vi "NI Read XLSX File.vi"(8 "error in":errorcluster, 11 "XLSX File":path) -> (0 "error out":errorcluster, 2 "Sheet Names":string[](array[string]), 3 "Sheet Data":cluster{"Array":string[][]}[](array[cluster]))   [LabVIEW 2018]
doc: "Reads all sheets from the specified <b>XLSX File</b>. This VI does <b>not</b> require Microsoft Excel to be installed.\n\nEach sheet is returned as a 2D Array of Strings. You will need to perform additional conversion if you require data in numeric format.\n\nTime data (date and/or time) is returned as a number of days elapsed since January 1, 1900. Hour/minute/second information will be returned as a fraction of a day (24 hours)."
uses:
  <vilib>/zip/NI_Unzip.lvlib
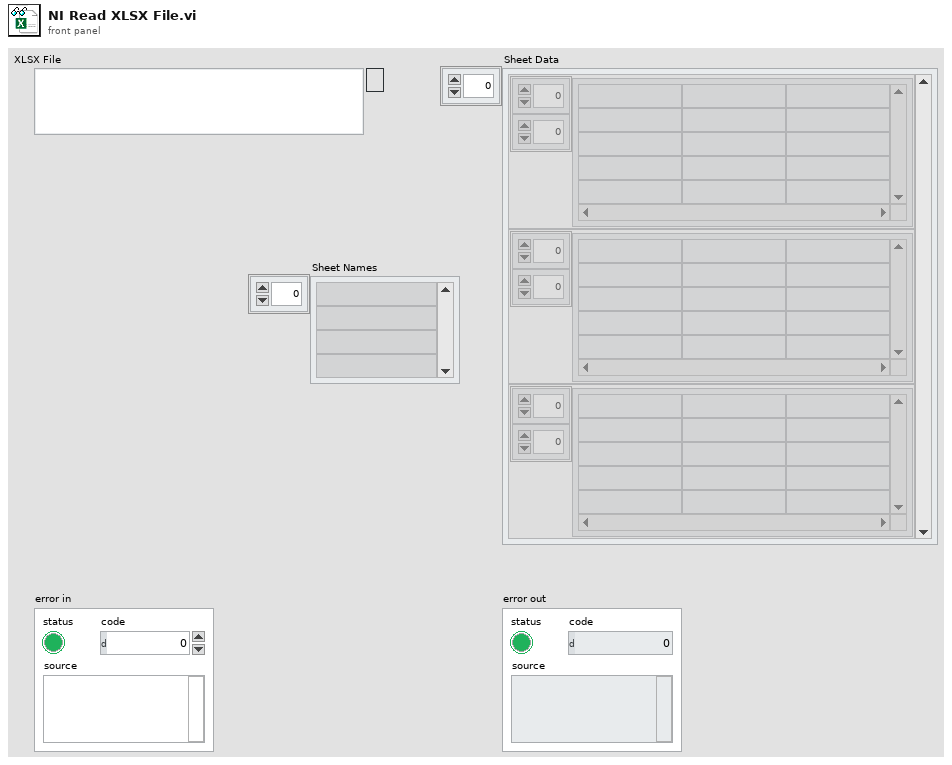
[diagram p1: front panel]
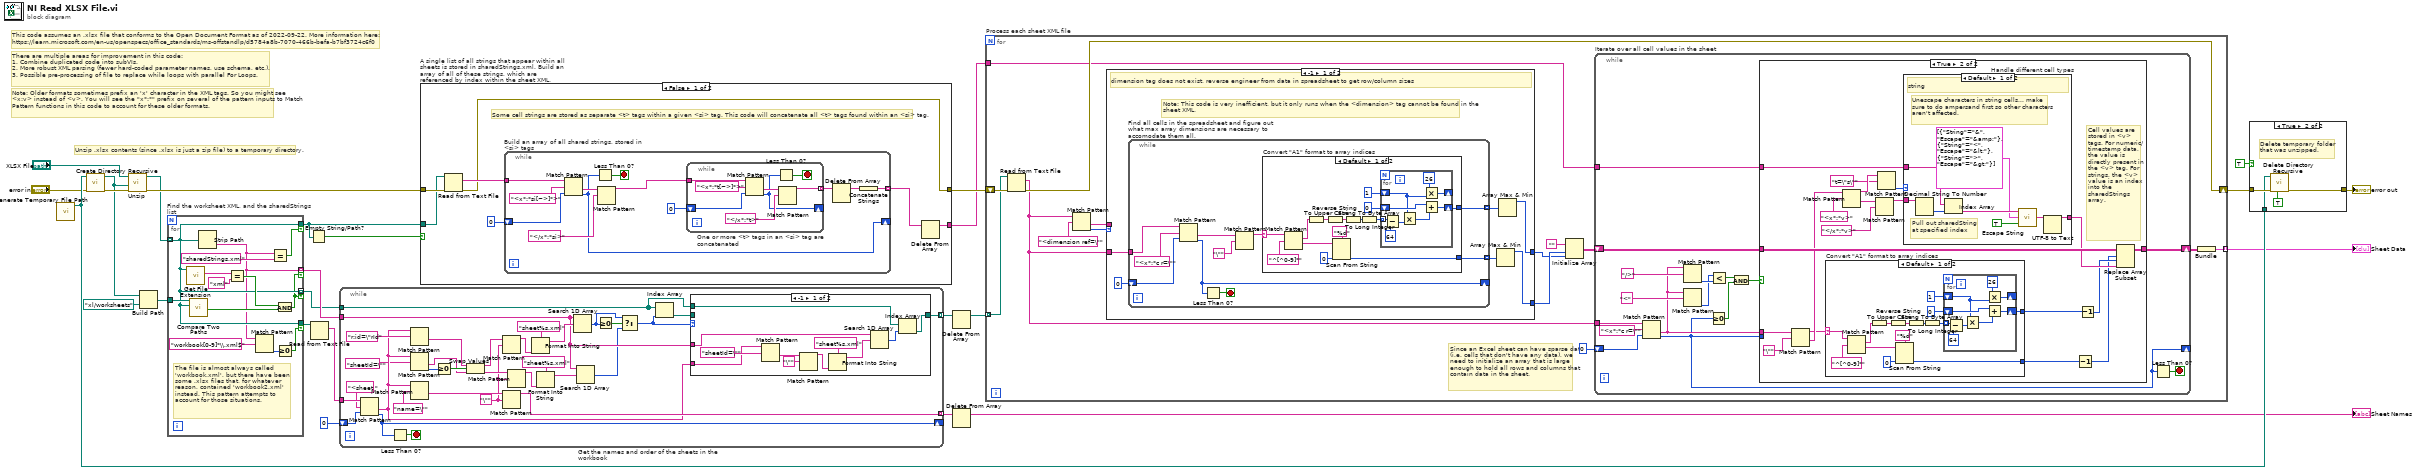
[diagram p0: block diagram]
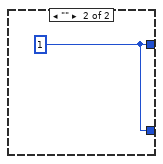
[diagram p5: hidden frame]
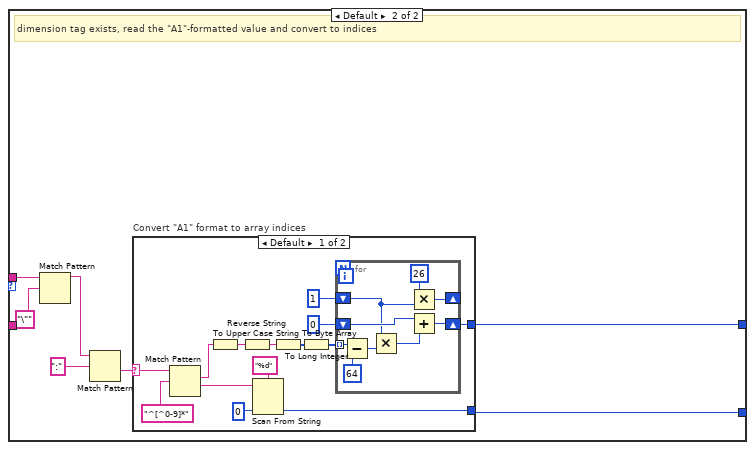
[diagram p6: hidden frame]
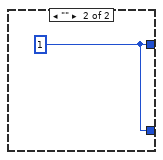
[diagram p7: hidden frame]
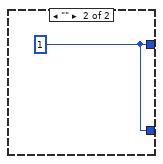
[diagram p9: hidden frame]
diagram:
  # "Note: Older formats sometimes prefix an 'x' character in the XML tags. So you might see <x:v> instead of <v>. You will see the \"x*:*\" prefix on several of the pattern inputs to Match Pattern functions in this code to account for these older formats."
  # "There are multiple areas for improvement in this code:\n1. Combine duplicated code into subVIs.\n2. More robust XML parsing (fewer hard-coded parameter names, use schema, etc.).\n3. Possible pre-processing of file to replace while loops with parallel For Loops."
  # "Unzip .xlsx contents (since .xlsx is just a zip file) to a temporary directory."
  # "This code assumes an .xlsx file that conforms to the Open Document Format as of 2022-09-22. More information here:\nhttps://learn.microsoft.com/en-us/openspecs/office_standards/ms-offstandlp/d5784a8b-7070-466b-befa-b7bf3724c6f0"
  n1 = call <vilib>:"Generate Temporary File Path.vi"() -> ("Unique Temporary File Path"=w16:path)  [unwired: 10 in, 1 out]
  n2 = call <vilib>:"Create Directory Recursive.vi"("error in (no error)"="error in", "directory"=w16) -> ("error out"=w26:errorcluster, "directory copy"=w19:path)  [unwired: 3 in, 1 out]
  n3 = call <vilib>:"Unzip.vi"("error in (no error)"=w26, "Target directory (same as Zip file if empty)"=w19, "Zip file"="XLSX File") -> ("error out"=w25:errorcluster, "Unzipped files"=w20:path[])  [unwired: 6 in, 1 out]
  n4 = Build Path(base path=w19, name or relative path=path "xl/worksheets") -> (appended path=w17:path)
  n5 = for "Find the worksheet XML, and the sharedStrings list" {
    tunnel: w20 -> [w32] mode=indexing
    tunnel: [w32] -> w13 if=w36
    tunnel: w17 -> [w38]
    tunnel: [w32] -> w7 mode=indexing if=w31
    tunnel: [w32] -> w11 if=w27
    tunnel: [w30] -> w8 mode=indexing if=w31
    # "The file is almost always called 'workbook.xml', but there have been some .xlsx files that, for whatever reason, contained 'workbook2.xml' instead. This pattern attempts to account for those situations."
    n6 = call <vilib>:"Get File Extension.vi"("file"=w32) -> ("lowercase file extension"=w35:string)  [unwired: 6 in, 4 out]
    n7 = call <vilib>:"Compare Two Paths.vi"("Path 2"=w32, "Path 1"=w38) -> ("Path 2 Relative to Path 1?"=w37:bool)  [unwired: 6 in, 3 out]
    n8 = Strip Path(path=w32) -> (name=w30:string)  [unwired: 1 out]
    n9 = Equal?(x=w35, y="xml") -> (x = y?=w33:bool)
    n10 = Match Pattern(string=w30, regular expression="workbook[0-9]*\\.xml$" ("y")) -> (offset past match=w28:i32)  [unwired: 1 in, 3 out]
    n11 = Equal?(x=w30, y="sharedStrings.xml") -> (x = y?=w36:bool)
    n12 = And(x=w33, y=w37) -> (x .and. y?=w31:bool)
    n13 = Greater Or Equal To 0?(x=w28) -> (x >= 0?=w27:bool)
  }
  n14 = Empty String/Path?(string/path=w13) -> (empty?=w12:bool)
  n15 = Read from Text File(file (use dialog)=w11) -> (text=w10:string)  [unwired: 3 in, 3 out]
  n16 = while "Get the names and order of the sheets in the workbook" {
    tunnel: w10 -> [w71]
    shift-right: [w69] -> _
    shift-left: 0 -> [w70]
    tunnel: [w63] -> w4 mode=indexing
    tunnel: w8 -> [w44]
    tunnel: w7 -> [w57]
    tunnel: [w59] -> w6 mode=indexing
    stop <- w67 stop-if-true
    w46 = "\"" ("regular expression")
    n17 = Match Pattern(string=w71, regular expression="<sheet ", offset (0)=w70) -> (after substring=w56:string, offset past match=w69:i32)  [unwired: 2 out]
    n18 = Less Than 0?(x=w69) -> (x < 0?=w67:bool)
    n19 = Match Pattern(string=w56, regular expression="r:id=\"rId") -> (after substring=w49:string)  [unwired: 1 in, 3 out]
    n20 = Match Pattern(string=w56, regular expression="name=\"") -> (after substring=w65:string)  [unwired: 1 in, 3 out]
    n21 = Match Pattern(string=w56, regular expression="sheetId=\"") -> (after substring=w50:string, offset past match=w54:i32)  [unwired: 1 in, 2 out]
    n22 = Greater Or Equal To 0?(x=w54) -> (x >= 0?=w51:bool)
    n23 = Swap Values(12:w49, 13:w51, 14:w50) -> (1:w48:string, 3:w47:string)
    n24 = Match Pattern(string=w48, regular expression=w46) -> (before substring=w62:string)  [unwired: 1 in, 3 out]
    n25 = Match Pattern(string=w65, regular expression=w46) -> (before substring=w63:string)  [unwired: 1 in, 3 out]
    n26 = Match Pattern(string=w47, regular expression=w46) -> (before substring=w52:string)  [unwired: 1 in, 3 out]
    n27 = Format Into String(format string="sheet%s.xml", w62) -> (resulting string=w60:string)  [unwired: 2 in, 1 out]
    n28 = Format Into String(format string="sheet%s.xml", w52) -> (resulting string=w45:string)  [unwired: 2 in, 1 out]
    n29 = Search 1D Array(1D array=w44, element=w60) -> (index of element=w42:i32)  [unwired: 1 in]
    n30 = Search 1D Array(1D array=w44, element=w45) -> (index of element=w41:i32)  [unwired: 1 in]
    n31 = Greater Or Equal To 0?(x=w42) -> (x >= 0?=w43:bool)
    n32 = Select(t=w42, s=w43, f=w41) -> (s? t:f=w40:i32)
    n33 = Index Array(array=w57, index=w40) -> (element=w58:path)
    n34 = case shown="-1" w40 {
      tunnel: [w76 w83] -> w59
      tunnel: w58 -> [_ w83]
      tunnel: w57 -> [w75 _]
      tunnel: w44 -> [w74 _]
      tunnel: w56 -> [w72 _]
      frame -1 {
        n35 = Match Pattern(string=w72, regular expression="sheetId=\"") -> (after substring=w81:string)  [unwired: 1 in, 3 out]
        n36 = Match Pattern(string=w81, regular expression="\"") -> (before substring=w80:string)  [unwired: 1 in, 3 out]
        n37 = Format Into String(format string="sheet%s.xml", w80) -> (resulting string=w78:string)  [unwired: 2 in, 1 out]
        n38 = Search 1D Array(1D array=w74, element=w78) -> (index of element=w77:i32)  [unwired: 1 in]
        n39 = Index Array(array=w75, index=w77) -> (element=w76:path)
      }
      frame Default {
      }
    }
  }
  n40 = case "A single list of all strings that appear within all sheets is stored in sharedStrings.xml. Build an array of all of these strings, which are referenced by index within the sheet XML." shown="False" w12 {
    tunnel: w25 -> [w90 w111]
    tunnel: [w85 w111] -> w24
    tunnel: w13 -> [w89 _]
    tunnel: [w86 _] -> w14
    frame False {
      # "Some cell strings are stored as separate <t> tags within a given <si> tag. This code will concatenate all <t> tags found within an <si> tag."
      n41 = Read from Text File(file (use dialog)=w89, error in=w90) -> (text=w88:string, error out=w85:errorcluster)  [unwired: 2 in, 2 out]
      n42 = while "Build an array of all shared strings, stored in <si> tags" {
        tunnel: w88 -> [w94]
        tunnel: [w99] -> w87 mode=indexing
        shift-right: [w93] -> _
        shift-left: 0 -> [w95]
        stop <- w91 stop-if-true
        n43 = Match Pattern(string=w94, regular expression="<x*:*si[~>]*>", offset (0)=w95) -> (after substring=w97:string, offset past match=w93:i32)  [unwired: 2 out]
        n44 = Less Than 0?(x=w93) -> (x < 0?=w91:bool)
        n45 = Match Pattern(string=w97, regular expression="</x*:*si>") -> (before substring=w92:string)  [unwired: 1 in, 3 out]
        n46 = while "One or more <t> tags in an <si> tag are concatenated" {
          tunnel: w92 -> [w110]
          tunnel: [w106] -> w102 mode=indexing
          shift-right: [w104] -> _
          shift-left: 0 ("offset past match") -> [w103]
          stop <- w105 stop-if-true
          n47 = Match Pattern(string=w110, regular expression="<x*:*t[~>]*>", offset (0)=w103) -> (after substring=w108:string, offset past match=w104:i32)  [unwired: 2 out]
          n48 = Less Than 0?(x=w104) -> (x < 0?=w105:bool)
          n49 = Match Pattern(string=w108, regular expression="</x*:*t>") -> (before substring=w106:string)  [unwired: 1 in, 3 out]
        }
        n50 = Delete From Array(array=w102) -> (array with subset deleted=w100:string[])  [unwired: 2 in, 1 out]
        n51 = Concatenate Strings(w100) -> (w99:string)
      }
      n52 = Delete From Array(array=w87) -> (array with subset deleted=w86:string[])  [unwired: 2 in, 1 out]
    }
    frame True {
      # "No sharedStrings.xml file within .xlsx."
    }
  }
  n53 = Delete From Array(array=w6) -> (array with subset deleted=w5:path[])  [unwired: 2 in, 1 out]
  n54 = Delete From Array(array=w4) -> (array with subset deleted=→"Sheet Names":string[])  [unwired: 2 in, 1 out]
  n55 = for "Process each sheet XML file" {
    shift-right: [w125] -> w23
    shift-left: w24 -> [w126]
    tunnel: w5 -> [w124] mode=indexing
    tunnel: [w118] -> w15 mode=indexing
    tunnel: w14 -> [w116]
    # "Since an Excel sheet can have sparse data (i.e. cells that don't have any data), we need to initialize an array that is large enough to hold all rows and columns that contain data in the sheet."
    n56 = Read from Text File(file (use dialog)=w124, error in=w126) -> (text=w112:string, error out=w125:errorcluster)  [unwired: 2 in, 2 out]
    n57 = Match Pattern(string=w112, regular expression="<dimension ref=\"") -> (after substring=w122:string, offset past match=w113:i32)  [unwired: 1 in, 2 out]
    n58 = case shown="-1" w113 {
      tunnel: w122 -> [_ w173]
      tunnel: [w129 w171] -> w115
      tunnel: [w127 w170] -> w114
      tunnel: w112 -> [w132 _]
      frame -1 {
        # "Note: This code is very inefficient, but it only runs when the <dimension> tag cannot be found in the sheet XML."
        # "dimension tag does not exist, reverse engineer from data in spreadsheet to get row/column sizes"
        n59 = while "Find all cells in the spreadsheet and figure out what max array dimensions are necessary to accomodate them all." {
          tunnel: w132 -> [w135]
          tunnel: [w137] -> w130 mode=indexing
          shift-right: [w133] -> _
          shift-left: 0 -> [w134]
          tunnel: [w136] -> w128 mode=indexing
          stop <- w142 stop-if-true
          n60 = Match Pattern(string=w135, regular expression="<x*:*c r=\"", offset (0)=w134) -> (after substring=w140:string, offset past match=w133:i32)  [unwired: 2 out]
          n61 = Less Than 0?(x=w133) -> (x < 0?=w142:bool)
          n62 = Match Pattern(string=w140, regular expression="\"") -> (before substring=w138:string)  [unwired: 1 in, 3 out]
          n63 = case "Convert \"A1\" format to array indices" shown="Default" w138 {
            selector: w138 -> [w147 _]
            tunnel: [w150 w166] -> w136
            tunnel: [w146 w166] -> w137
            frame Default {
              n64 = Match Pattern(string=w147, regular expression="^[^0-9]*") -> (match substring=w149:string, after substring=w156:string)  [unwired: 1 in, 2 out]
              n65 = To Upper Case(1:w149) -> (0:w151:string)
              n66 = Reverse String(1:w151) -> (0:w153:string)
              n67 = Scan From String(format string="%d" ("Format String"), input string=w156, default 1=0) -> (output 1=w146:i32)  [unwired: 2 in, 3 out]
              n68 = String To Byte Array(string=w153) -> (unsigned byte array=w152:u8[])
              n69 = To Long Integer(number=w152) -> (32bit integer=w148:i32[])
              n70 = for {
                tunnel: w148 -> [w165] mode=indexing
                shift-right: [w163] -> w150
                shift-left: 0 -> [w160]
                shift-right: [w164] -> _
                shift-left: 1 -> [w159]
                n71 = Subtract(x=w165, y=64) -> (x-y=w161:i32)
                n72 = Multiply(x=w159, y=w161) -> (x*y=w162:i32)
                n73 = Multiply(x=26, y=w159) -> (x*y=w164:i32)
                n74 = Add(x=w160, y=w162) -> (x+y=w163:i32)
              }
            }
            frame "" {
              w166 = 1
            }
          }
        }
        n75 = Array Max & Min(array=w130) -> (max value=w129:i32)  [unwired: 3 out]
        n76 = Array Max & Min(array=w128) -> (max value=w127:i32)  [unwired: 3 out]
      }
      frame Default {
        # "Code copied from:\n[LabVIEW 20xx]\\vi.lib\\addons\\_office\\excel.llb\\Excel Get Excel Location.vi"
        # "dimension tag exists, read the \"A1\"-formatted value and convert to indices"
        n77 = Match Pattern(string=w173, regular expression="\"") -> (before substring=w169:string)  [unwired: 1 in, 3 out]
        n78 = Match Pattern(string=w169, regular expression=":") -> (after substring=w167:string)  [unwired: 1 in, 3 out]
        n79 = case "Convert \"A1\" format to array indices" shown="Default" w167 {
          selector: w167 -> [w178 _]
          tunnel: [w181 w197] -> w170
          tunnel: [w177 w197] -> w171
          frame Default {
            n80 = Match Pattern(string=w178, regular expression="^[^0-9]*") -> (match substring=w180:string, after substring=w187:string)  [unwired: 1 in, 2 out]
            n81 = To Upper Case(1:w180) -> (0:w182:string)
            n82 = Reverse String(1:w182) -> (0:w184:string)
            n83 = Scan From String(format string="%d" ("Format String"), input string=w187, default 1=0) -> (output 1=w177:i32)  [unwired: 2 in, 3 out]
            n84 = String To Byte Array(string=w184) -> (unsigned byte array=w183:u8[])
            n85 = To Long Integer(number=w183) -> (32bit integer=w179:i32[])
            n86 = for {
              tunnel: w179 -> [w196] mode=indexing
              shift-right: [w194] -> w181
              shift-left: 0 -> [w191]
              shift-right: [w195] -> _
              shift-left: 1 -> [w190]
              n87 = Subtract(x=w196, y=64) -> (x-y=w192:i32)
              n88 = Multiply(x=w190, y=w192) -> (x*y=w193:i32)
              n89 = Multiply(x=26, y=w190) -> (x*y=w195:i32)
              n90 = Add(x=w191, y=w193) -> (x+y=w194:i32)
            }
          }
          frame "" {
            w197 = 1
          }
        }
      }
    }
    n91 = Initialize Array("", w115, w114) -> (w120:string[][])
    n92 = while "Iterate over all cell values in the sheet" {
      shift-right: [w209] -> w119
      shift-left: w120 -> [w208]
      tunnel: w112 -> [w213]
      shift-right: [w201] -> _
      shift-left: 0 -> [w211]
      tunnel: w116 -> [w207]
      stop <- w210 stop-if-true
      n93 = Match Pattern(string=w213, regular expression="<x*:*c r=\"", offset (0)=w211) -> (after substring=w203:string, offset past match=w201:i32)  [unwired: 2 out]
      n94 = Match Pattern(string=w203, regular expression="/>") -> (offset past match=w204:i32)  [unwired: 1 in, 3 out]
      n95 = Match Pattern(string=w203, regular expression="<") -> (offset past match=w202:i32)  [unwired: 1 in, 3 out]
      n96 = Greater Or Equal To 0?(x=w201) -> (x >= 0?=w199:bool)
      n97 = Less?(x=w202, y=w204) -> (x < y?=w200:bool)
      n98 = And(x=w200, y=w199) -> (x .and. y?=w198:bool)
      n99 = case shown="True" w198 {
        tunnel: w203 -> [_ w233]
        tunnel: [w214 w230] -> w209
        tunnel: w208 -> [w214 w231]
        tunnel: w207 -> [_ w220]
        tunnel: w201 -> [_ _]
        frame False {
          # "No more cells found in the sheet XML. Stop the loop."
        }
        frame True {
          # "Cell values are stored in <v> tags. For numeric/timestamp data, the value is directly present in the <v> tag. For strings, the <v> value is an index into the sharedStrings array."
          n100 = Match Pattern(string=w233, regular expression="\"") -> (before substring=w217:string, after substring=w226:string)  [unwired: 1 in, 2 out]
          n101 = case "Convert \"A1\" format to array indices" shown="Default" w217 {
            selector: w217 -> [w238 _]
            tunnel: [w241 w257] -> w216
            tunnel: [w237 w257] -> w215
            frame Default {
              n102 = Match Pattern(string=w238, regular expression="^[^0-9]*") -> (match substring=w240:string, after substring=w247:string)  [unwired: 1 in, 2 out]
              n103 = To Upper Case(1:w240) -> (0:w242:string)
              n104 = Reverse String(1:w242) -> (0:w244:string)
              n105 = Scan From String(format string="%d" ("Format String"), input string=w247, default 1=0) -> (output 1=w237:i32)  [unwired: 2 in, 3 out]
              n106 = String To Byte Array(string=w244) -> (unsigned byte array=w243:u8[])
              n107 = To Long Integer(number=w243) -> (32bit integer=w239:i32[])
              n108 = for {
                tunnel: w239 -> [w256] mode=indexing
                shift-right: [w254] -> w241
                shift-left: 0 -> [w251]
                shift-right: [w255] -> _
                shift-left: 1 -> [w250]
                n109 = Subtract(x=w256, y=64) -> (x-y=w252:i32)
                n110 = Multiply(x=w250, y=w252) -> (x*y=w253:i32)
                n111 = Multiply(x=26, y=w250) -> (x*y=w255:i32)
                n112 = Add(x=w251, y=w253) -> (x+y=w254:i32)
              }
            }
            frame "" {
              w257 = 1
            }
          }
          n113 = Match Pattern(string=w226, regular expression="<x*:*v>") -> (before substring=w225:string, after substring=w228:string)  [unwired: 1 in, 2 out]
          n114 = Match Pattern(string=w228, regular expression="</x*:*v>") -> (before substring=w221:string)  [unwired: 1 in, 3 out]
          n115 = Match Pattern(string=w225, regular expression="t=\"s\"") -> (offset past match=w223:i32)  [unwired: 1 in, 3 out]
          n116 = case "Handle different cell types" shown="Default" w223 {
            tunnel: [w258 w266] -> w222
            tunnel: w221 -> [w265 w266]
            tunnel: w220 -> [w263 _]
            frame Default {
              # "Unescape characters in string cells... make sure to do ampersand first so other characters aren't affected."
              # "Pull out sharedString at specified index"
              # "string"
              n117 = Decimal String To Number(string=w265) -> (number=w264:i32)  [unwired: 2 in, 1 out]
              n118 = Index Array(array=w263, index=w264) -> (element=w261:string)
              n119 = call <vilib>:"Escape String.vi"("Remove Escapes? (False)"=TRUE, "Escapes"=cluster{"String":string, "Escape":string}[] [{"String"="&", "Escape"="&amp;"}, {"String"="<", "Escape"="&lt;"}, {"String"=">", "Escape"="&gt;"}], "String in"=w261) -> ("String out"=w259:string)
              n120 = UTF-8 to Text(11:w259) -> (3:w258:string)  [unwired: 2 in, 1 out]
            }
            frame -1 {
              # "Use <v> value"
              # "number/time stamp"
            }
          }
          n121 = Decrement(x=w215) -> (x-1=w218:i32)
          n122 = Decrement(x=w216) -> (x-1=w219:i32)
          n123 = Replace Array Subset(array=w231, new element=w222, index (row)=w218, index (col)=w219) -> (w230:string[][])
        }
      }
      n124 = Less Than 0?(x=w201) -> (x < 0?=w210:bool)
    }
    n125 = Bundle(w119) -> (w118:cluster{string[][]})  [unwired: 1 in]
  }
  "Sheet Data" <- w15
  n126 = case shown="True" TRUE {
    tunnel: w23 -> [w267 w271]
    tunnel: [w267 w270] -> w22
    tunnel: w16 -> [_ w269]
    frame False {
      # "Keep temporary unzip files for debugging"
    }
    frame True {
      # "Delete temporary folder that was unzipped."
      n127 = call <vilib>:"Delete Directory Recursive.vi"("keep deleting on error? (F)"=TRUE, "error in (no error)"=w271, "Folder to Delete"=w269) -> ("error out"=w270:errorcluster)  [unwired: 7 in, 1 out]
    }
  }
  "error out" <- w22
